vi "Entrain.vi"() -> ()   [LabVIEW 2012]
uses:
  <vilib>/Analysis/3filter.llb/Filter Passband Type.ctl
  Treatment.ctl
  Treatment type.ctl
  Data.ctl
  <vilib>/Platform/TimedLoop/XDataNode/timing_clust.ctl
  <vilib>/Platform/TimedLoop/XDataNode/nitl_modes.ctl
  <vilib>/Platform/TimedLoop/XDataNode/wakeup.ctl
  <vilib>/Platform/TimedLoop/XDataNode/XDataNode.xnode
  <vilib>/Platform/TimedLoop/XDataNode/XDNodeRunTimeDep.lvlib
  <vilib>/Analysis/NI_AALBase.lvlib
panel:
  out "R":dbl[](array[numeric])
  out "mean phase":dbl[](array[numeric])
  in  "reset phase":bool
  in  "enable":bool=TRUE caption="Enable motor"
  out "Cur freq":dbl caption="Stimulus frequency (Hz)"
  out "PSD":cluster{"f0":dbl, "df":dbl, "magnitude":dbl[]}[](graph)
  in  "Threshold":dbl=0.1
  out "Sweep":cluster{cluster{dbl, dbl}[]}[](graph)
  out "Raw data":waveform(dbl)[](graph)
  in  "Stop":bool
  in  "Go":bool
  in  "Treatment type":T1(tab)
  in  "Duration":dbl=inf min=0.0 step=1.0
  in  "Noise":dbl min=0.0 step=0.5
  in  "Frequency":dbl=1.0 min=0.0 step=0.05
  in  "Amplitude":dbl=30.0 min=0.0 step=1.0
  in  "Dur unit":enum16{"sec", "cycles"}(ring)
  in  "noise filter type":T2=enum."Bandpass"
  in  "Lo freq cutoff":dbl min=0.0 step=0.5
  in  "Hi freq cutoff":dbl min=0.0 step=0.5
  in  "End noise":dbl caption="End" min=0.0 step=0.5
  in  "End amplitude":dbl=30.0 caption="End" min=0.0 step=1.0
  in  "Start amp":dbl=30.0 caption="Start" min=0.0 step=1.0
  in  "Frequency":dbl=1.0 min=0.0 step=0.05
  in  "Start noise":dbl caption="Start" min=0.0 step=0.5
  in  "Lo freq cutoff 3":dbl caption="Lo freq cutoff" min=0.0 step=0.5
  in  "Hi freq cutoff 3":dbl caption="Hi freq cutoff" min=0.0 step=0.5
  in  "noise filter type 4":T2=enum."Bandpass" caption="Noise filter type"
  in  "Duration":dbl=inf min=0.0 step=1.0
  in  "Dur unit 4":enum16{"sec", "cycles"}(ring)
  in  "End freq":dbl=1.0 caption="End frequency" min=0.0 step=0.05
  in  "Duration":dbl=inf min=0.0 step=1.0
  in  "Noise":dbl min=0.0 step=0.5
  in  "Start freq":dbl=1.0 caption="Start frequency" min=0.0 step=0.05
  in  "Amp":dbl=30.0 caption="Amplitude" min=0.0 step=1.0
  in  "noise filter type 2":T2=enum."Bandpass" caption="Noise filter type"
  in  "Lo freq cutoff":dbl min=0.0 step=0.5
  in  "Hi freq cutoff":dbl min=0.0 step=0.5
  in  "Frequency 2":dbl=1.0 min=0.0 step=0.05
  in  "Amplitude 2":dbl=30.0 min=0.0 step=1.0
  in  "Duration":dbl=inf min=0.0 step=1.0
  in  "Frequency 1":dbl=1.0 min=0.0 step=0.05
  in  "Amplitude 1":dbl=30.0 min=0.0 step=1.0
  in  "Dur unit 2":enum16{"sec", "cycles"}(ring)
  out "Data file":path
  # "deg"
  # "Hz"
  # "deg"
  # "Hz"
  # "Hz"
  # "Noise is approximately\n4x lower than specified"
  # "Amplitude:"
  # "deg"
  # "Hz"
  # "deg"
  # "Hz"
  # "Hz"
  # "Send the position\nto zero"
  # "deg"
  # "Hz"
  # "Hz"
  # "deg"
  # "sec"
  # "deg"
  # "Hz"
  # "deg"
  # "Hz"
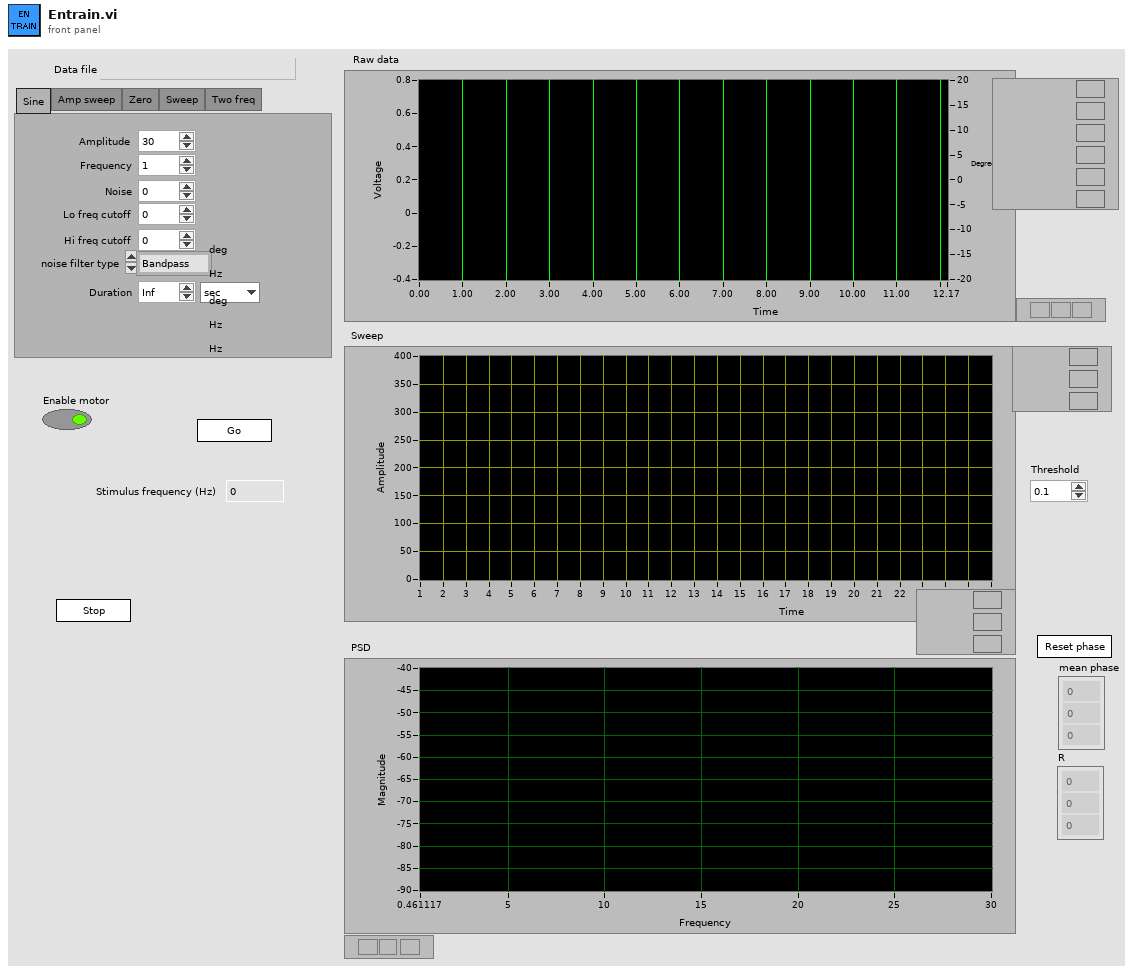
[diagram p1: front panel]
types:
  T1 = enum32{"Sine", "Amp sweep", "Zero", "Sweep", "Two freq"}
  T2 = typedef "NI_AALBase.lvlib/Filter Passband Type.ctl" = enum32{"Lowpass", "Highpass", "Bandpass", "Bandstop"}
  T3 = typedef "Treatment.ctl" = cluster{"sample":dbl, "startphase":dbl, "type":T4, "frequency":dbl, "amplitude":dbl, "noise":dbl, "duration":dbl, "kfreq":dbl, "noisehifreq":dbl, "frequency2":dbl, "amplitude2":dbl, "startphase2":dbl, "noise filter type":T2, "noiselofreq":dbl, "amp change":dbl, "noise change":dbl}
  T4 = typedef "Treatment type.ctl" = enum16{"Zero", "Sine", "Frequency sweep", "Two frequency"}
  T5 = typedef "Sampling info.ctl" = cluster{"Channels":T6[], "Sampling freq":i32, "Output freq":i32, "Update freq":i32, "Steps per rev":i32, "Counts per rev":i32, "Amplifier":string, "Motor driver":string, "Step bit":u8, "Max speed":dbl, "Max accel":dbl, "Pos gain":dbl, "Vel gain":dbl}
  T6 = typedef "Channel.ctl" = cluster{"Name":string, "Chan":tag, "Gain":u16, "Lo cutoff":dbl, "Hi cutoff":dbl, "Notch":bool}
  T7 = typedef "Data.ctl" = cluster{"Voltage data":dbl[][], "Encoder data":dbl[], "Motor output":dbl[], "Current treatment":T3, "Motor speed":dbl[], "Clipped motor":dbl[], "new treatment":bool}
  T8 = typedef "File refs.ctl" = cluster{"file":T9, "voltage data":i32, "motor data":i32, "command data":i32, "encoder data":i32}
  T9 = typedef "hid_t.ctl" = i32
  T10 = typedef "Run info.ctl" = cluster{"voltage task":refnum<k21>, "dummy output task":refnum<k21>, "digital output task":refnum<k21>, "encoder task":refnum<k21>, "n input samples":i32, "n output samples":i32, "max speed":dbl, "max accel":dbl, "last pos":dbl, "last vel":dbl, "pos gain":dbl, "vel gain":dbl, "input dt":dbl}
  T11 = typedef "XDNodeRunTimeDep.lvlib/timing_clust.ctl" = cluster{"Expected End [f-1]":u64, "Actual End [f-1]":u64, "Finished Late? [f-1]":bool, "Expected End [i-1]":u64, "Actual End [i-1]":u64, "Finished Late? [i-1]":bool, "Expected Start [i]":u64, "Actual Start [i]":u64, "Expected Start [f]":u64, "Actual Start [f]":u64, "Source Name":string, "Structure Name":string, "Period":i64, "Deadline":i64, "Offset":i64, "Start":i64, "Priority":i32, "Timeout":i32, "Mode":T12, "Wakeup Reason":T13, "Error":errorcluster, "Source Type":string, "Secondary Source Type":string, "Global End Time":u64, "Global Start Time":u64, "Frame Duration":u64, "Iteration Duration":u64, "Assigned CPU":i32, "I/O Scan Engine Mode":u32}
  T12 = typedef "XDNodeRunTimeDep.lvlib/nitl_modes.ctl" = enum32{"No Change", "Process missed periods, maintain original phase", "Discard missed periods, maintain original phase", "Process missed periods, ignore original phase", "Discard missed periods, ignore original phase"}
  T13 = typedef "XDNodeRunTimeDep.lvlib/wakeup.ctl" = enum32{"Normal", "Aborted", "Asynchronous wakeup", "Timing source error", "Timed loop error", "Timeout"}
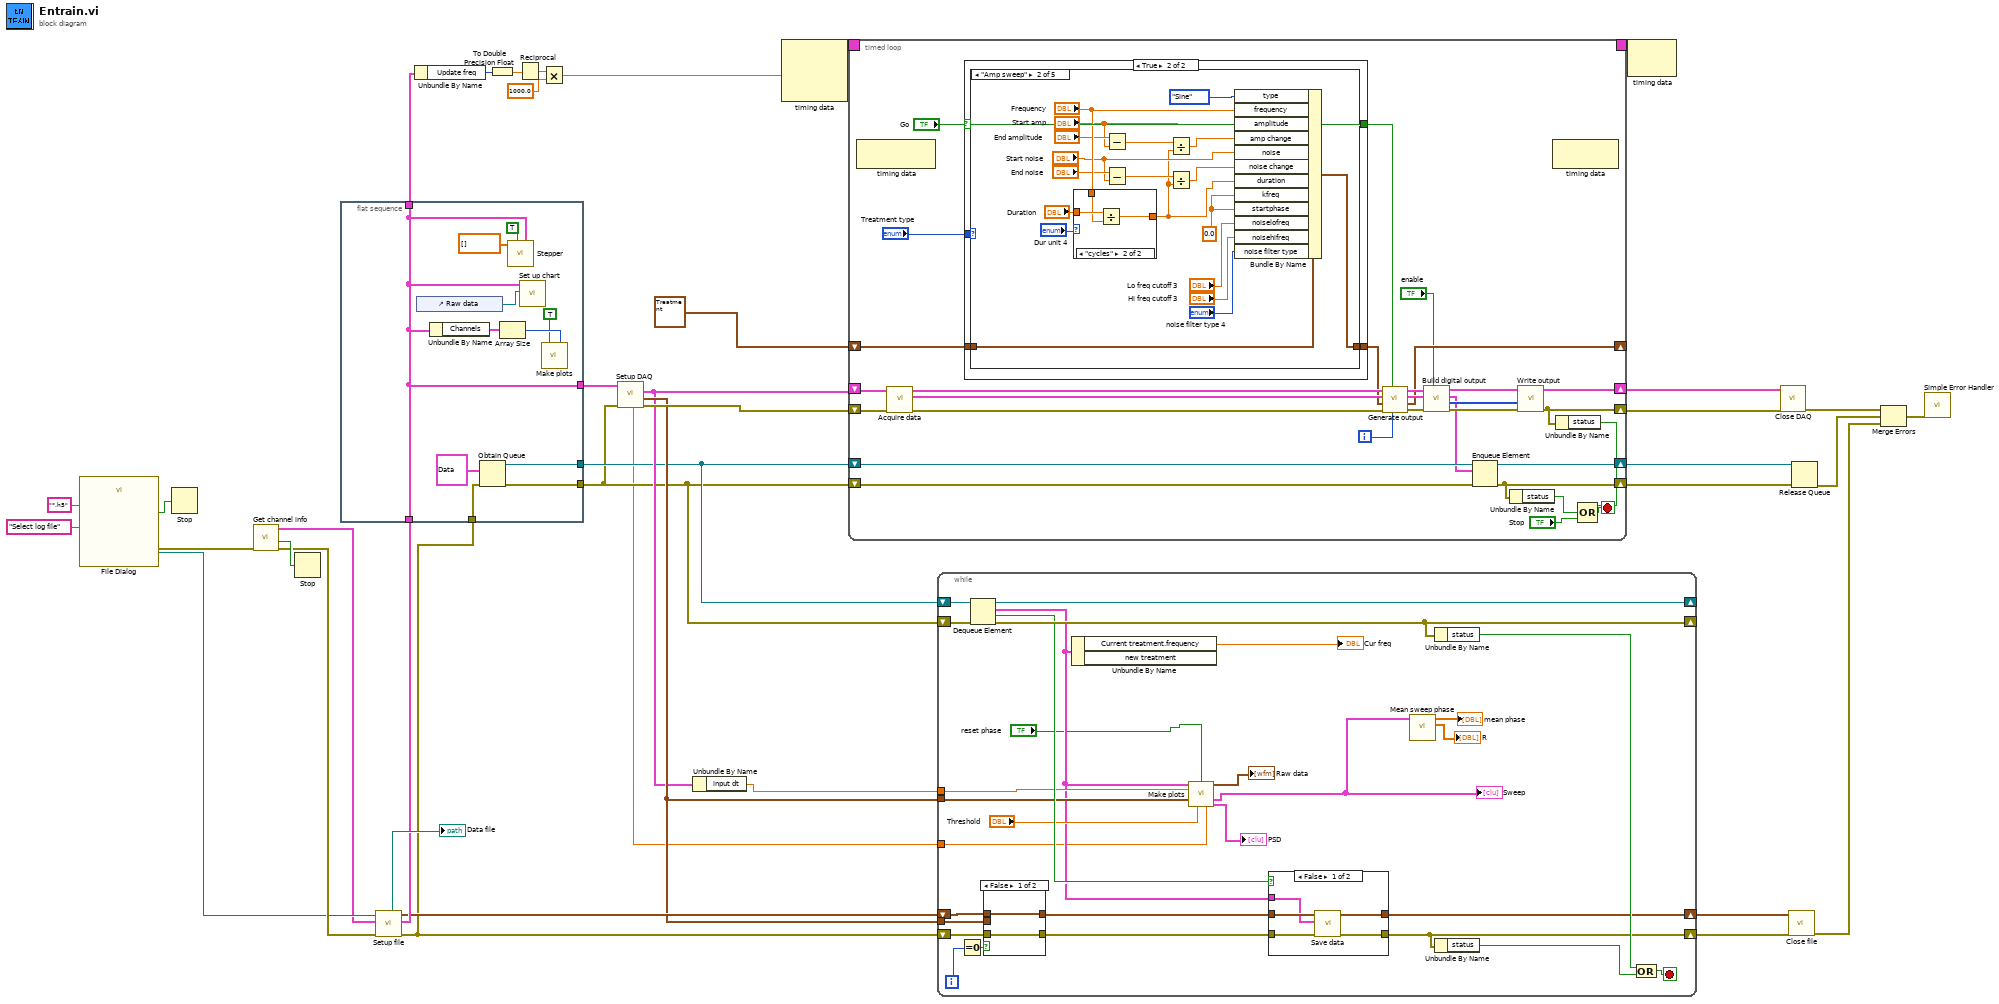
[diagram p0: block diagram]
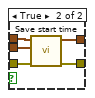
[diagram p2: hidden frame]
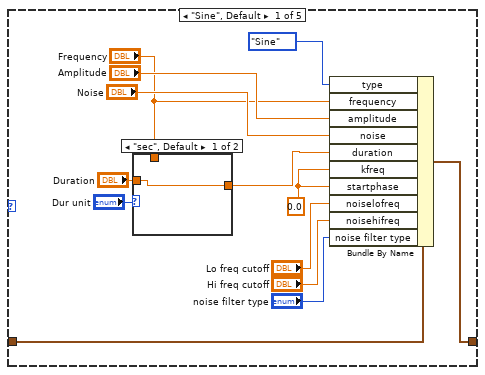
[diagram p5: hidden frame]
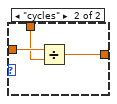
[diagram p6: hidden frame]
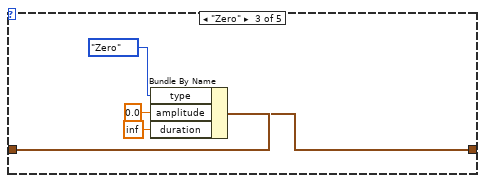
[diagram p8: hidden frame]
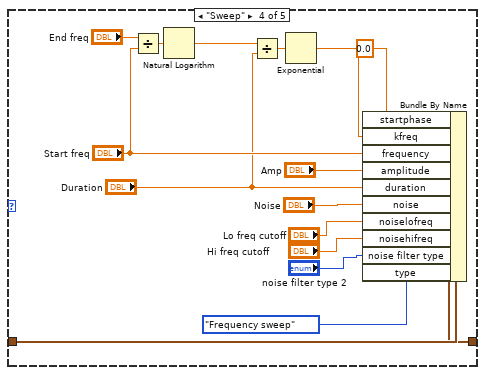
[diagram p9: hidden frame]
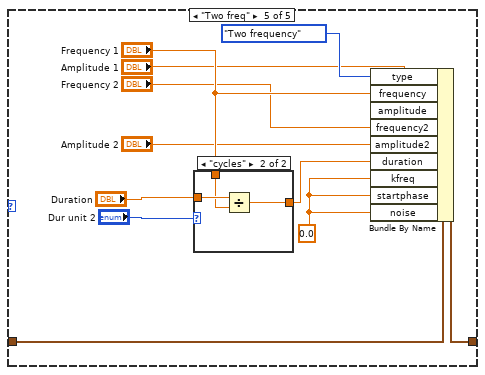
[diagram p10: hidden frame]
diagram:
  n1 = call "File Dialog"("prompt"="Select log file", "pattern (all files)"="*.h5") -> ("selected path"=w34:path, "cancelled"=w37:bool, "error out"=w33:errorcluster)  [unwired: 10 in, 1 out]
  n2 = Stop(stop? (T)=w37) -> ()
  n3 = call "Get channel info.vi"("error in"=w33) -> ("error out"=w35:errorcluster, "Cancelled"=w36:bool, "Sampling info"=w32:T5)  [unwired: 8 in]
  n4 = Stop(stop? (T)=w36) -> ()
  n5 = flat-sequence {
    tunnel: [w48] -> w3
    tunnel: w11 -> [w40]
    tunnel: [w42] -> w2
    tunnel: w9 -> [w41]
    tunnel: [w40] -> w7
    tunnel: [w40] -> w6
    frame #0 {
      n6 = control-ref of="Raw data"() -> (w46:refnum<vi>)
      n7 = Unbundle By Name(w40) -> ("Channels"=w45:T6[])
      n8 = Obtain Queue(element data type=T7 {"Voltage data"=[], "Encoder data"=[], "Motor output"=[], "Current treatment"={"sample"=0.0, "startphase"=0.0, "type"=enum."Zero", "frequency"=0.0, "amplitude"=0.0, "noise"=0.0, "duration"=0.0, "kfreq"=0.0, "noisehifreq"=0.0, "frequency2"=0.0, "amplitude2"=0.0, "startphase2"=0.0, "noise filter type"=enum."Lowpass", "noiselofreq"=0.0, "amp change"=0.0, "noise change"=0.0}, "Motor speed"=[], "Clipped motor"=[], "new treatment"=FALSE} ("Data"), error in (no error)=w41) -> (queue out=w48:refnum<queue>, error out=w42:errorcluster)  [unwired: 3 in, 1 out]
      n9 = Array Size(array=w45) -> (size(s)=w44:i32)
      n10 = call "Stepper.vi"("Sampling info"=w40, "initialize"=TRUE, "position"=dbl[] []) -> ()  [unwired: 7 in, 2 out]
      n11 = call "Set up chart.vi"("chart reference"=w46, "Sampling data"=w40) -> ()  [unwired: 10 in]
      n12 = call "Make plots.vi"("init"=TRUE, "nchan"=w44) -> ()  [unwired: 11 in, 3 out]
    }
  }
  n13 = call "Setup file.vi"("error in (no error)"=w35, "Sampling data"=w32, "selected path"=w34) -> ("error out"=w9:errorcluster, "Sampling data out"=w11:T5, "file refs"=w10:T8, "path out"=→"Data file":path)  [unwired: 5 in]
  n14 = Unbundle By Name(w7) -> ("Update freq"=w29:i32)
  n15 = To Double Precision Float(number=w29) -> (double precision float=w28:dbl)
  n16 = Reciprocal(x=w28) -> (1/x=w27:dbl)
  n17 = Multiply(x=w27, y=1000.0) -> (x*y=w14:dbl)
  n18 = call "Setup DAQ.vi"("error in (no error)"=w2, "Sampling info in"=w6) -> ("error out"=w13:errorcluster, "start time"=w8:timestamp, "Run info"=w4:T10, "output delay"=w1:dbl)  [unwired: 5 in, 1 out]
  n19 = Unbundle By Name(w4) -> ("input dt"=w12:dbl)
  n20 = node-c288(w14) -> (w31:T11)  [unwired: 2 in]
  n21 = timed-loop {
    timing: w31 -> [_]
    timing-out: [_] -> w30
    shift-right: [w58] -> _
    shift-left: T3 {"sample"=0.0, "startphase"=0.0, "type"=enum."Zero", "frequency"=0.0, "amplitude"=0.0, "noise"=0.0, "duration"=inf, "kfreq"=0.0, "noisehifreq"=20.0, "frequency2"=0.0, "amplitude2"=0.0, "startphase2"=0.0, "noise filter type"=enum."Lowpass", "noiselofreq"=0.0, "amp change"=0.0, "noise change"=0.0} ("Current treatment") -> [w54]
    shift-right: [w72] -> w17
    shift-left: w13 -> [w79]
    shift-right: [w71] -> w23
    shift-left: w2 -> [w74]
    shift-right: [w73] -> w16
    shift-left: w4 -> [w80]
    shift-right: [w66] -> w24
    shift-left: w3 -> [w75]
    i -> [w59]
    stop <- w68 stop-if-true
    n22 = node-c288() -> ()  [unwired: 1 in, 1 out]
    n23 = call "Acquire data.vi"("error in"=w79, "Run info"=w80) -> ("error out"=w76:errorcluster, "Data out"=w77:T7, "Run info out"=w78:T10)  [unwired: 7 in]
    n24 = case shown="True" "Go" {
      selector: "Go" -> [w81 w83]
      tunnel: "Treatment type" -> [_ w86]
      tunnel: w54 -> [w82 w85]
      tunnel: [w82 w84] -> w53
      tunnel: [w81 w83] -> w52
      frame False {
      }
      frame True {
        n25 = case shown="\"Amp sweep\"" w86 {
          tunnel: w85 -> [w93 w119 w128 w139 w154]
          tunnel: [w92 w118 w127 w138 w149] -> w84
          frame "Sine", Default {
            w90 = 0.0 ("kfreq")
            n26 = case shown="\"sec\", Default" "Dur unit" {
              tunnel: "Duration" -> [w100 w103]
              tunnel: "Frequency" -> [_ w102]
              tunnel: [w100 w101] -> w94
              frame "sec", Default {
              }
              frame "cycles" {
                n27 = Divide(x=w103, y=w102) -> (x/y=w101:dbl)
              }
            }
            n28 = Bundle By Name(cluster=w93, "type"=Treatment_type."Sine", "frequency"="Frequency", "amplitude"="Amplitude", "noise"="Noise", "duration"=w94, "kfreq"=w90, "startphase"=w90, "noiselofreq"="Lo freq cutoff", "noisehifreq"="Hi freq cutoff", "noise filter type"="noise filter type") -> (w92:T3)
          }
          frame "Amp sweep" {
            w116 = 0.0 ("kfreq")
            n29 = case shown="\"cycles\"" "Dur unit 4" {
              tunnel: "Duration" -> [w123 w126]
              tunnel: "Frequency" -> [_ w125]
              tunnel: [w123 w124] -> w105
              frame "sec", Default {
              }
              frame "cycles" {
                n30 = Divide(x=w126, y=w125) -> (x/y=w124:dbl)
              }
            }
            n31 = Subtract(x="End amplitude", y="Start amp") -> (x-y=w110:dbl)
            n32 = Subtract(x="End noise", y="Start noise") -> (x-y=w106:dbl)
            n33 = Divide(x=w110, y=w105) -> (x/y=w109:dbl)
            n34 = Divide(x=w106, y=w105) -> (x/y=w104:dbl)
            n35 = Bundle By Name(cluster=w119, "type"=Treatment_type."Sine", "frequency"="Frequency", "amplitude"="Start amp", "amp change"=w109, "noise"="Start noise", "noise change"=w104, "duration"=w105, "kfreq"=w116, "startphase"=w116, "noiselofreq"="Lo freq cutoff 3", "noisehifreq"="Hi freq cutoff 3", "noise filter type"="noise filter type 4") -> (w118:T3)
          }
          frame "Zero" {
            n36 = Bundle By Name(cluster=w128, "type"=Treatment_type."Zero", "amplitude"=0.0, "duration"=inf) -> (w127:T3)
          }
          frame "Sweep" {
            n37 = Divide(x="End freq", y="Start freq") -> (x/y=w147:dbl)
            n38 = Natural Logarithm(1:w147) -> (0:w146:dbl)
            n39 = Divide(x=w146, y="Duration") -> (x/y=w145:dbl)
            n40 = Exponential(1:w145) -> (0:w144:dbl)
            n41 = Bundle By Name(cluster=w139, "startphase"=0.0, "kfreq"=w144, "frequency"="Start freq", "amplitude"="Amp", "duration"="Duration", "noise"="Noise", "noiselofreq"="Lo freq cutoff", "noisehifreq"="Hi freq cutoff", "noise filter type"="noise filter type 2", "type"=Treatment_type."Frequency sweep") -> (w138:T3)
          }
          frame "Two freq" {
            w148 = 0.0 ("kfreq")
            n42 = case shown="\"cycles\"" "Dur unit 2" {
              tunnel: "Duration" -> [w159 w162]
              tunnel: "Frequency 1" -> [_ w161]
              tunnel: [w159 w160] -> w158
              frame "sec", Default {
              }
              frame "cycles" {
                n43 = Divide(x=w162, y=w161) -> (x/y=w160:dbl)
              }
            }
            n44 = Bundle By Name(cluster=w154, "type"=Treatment_type."Two frequency", "frequency"="Frequency 1", "amplitude"="Amplitude 1", "frequency2"="Frequency 2", "amplitude2"="Amplitude 2", "duration"=w158, "kfreq"=w148, "startphase"=w148, "noise"=w148) -> (w149:T3)
          }
        }
      }
    }
    n45 = call "Generate output.vi"("index"=w59, "new treatment"=w52, "error in"=w76, "Current treatment"=w53, "Data in"=w77, "Run info"=w78) -> ("error out"=w60:errorcluster, "Current treatment out"=w58:T3, "Data out"=w65:T7, "Run info out"=w63:T10)  [unwired: 2 in]
    n46 = call "Build digital output.vi"("enable"="enable", "error in"=w60, "Data in"=w65, "Run info"=w63) -> ("error out"=w61:errorcluster, "motor cmd"=w64:u32[], "Data out"=w57:T7, "Run info out"=w62:T10)  [unwired: 4 in]
    n47 = Enqueue Element(queue=w75, element=w57, error in (no error)=w74) -> (queue out=w66:refnum<queue>, error out=w71:errorcluster)  [unwired: 1 in, 1 out]
    n48 = Unbundle By Name(w71) -> ("status"=w69:bool)
    n49 = call "Write output.vi"("error in"=w61, "data"=w64, "Run info"=w62) -> ("error out"=w72:errorcluster, "Run info out"=w73:T10)  [unwired: 7 in]
    n50 = node-c288() -> ()  [unwired: 1 in, 1 out]
    n51 = Unbundle By Name(w72) -> ("status"=w70:bool)
    n52 = Compound Arithmetic op=OR(w70, w69, "Stop") -> (w68:bool)
  }
  n53 = while {
    shift-right: [w193] -> _
    shift-left: w2 -> [w187]
    shift-right: [w186] -> w22
    shift-left: w10 -> [w176]
    shift-right: [w185] -> w21
    shift-left: w9 -> [w174]
    shift-right: [w189] -> _
    shift-left: w3 -> [w188]
    tunnel: w8 -> [w183]
    tunnel: w12 -> [w181]
    tunnel: w8 -> [w179]
    tunnel: w1 -> [w169]
    i -> [w178]
    stop <- w192 stop-if-true
    n54 = Equal To 0?(x=w178) -> (x = 0?=w177:bool)
    n55 = Dequeue Element(queue=w188, error in (no error)=w187) -> (queue out=w189:refnum<queue>, element=w171:T7, timed out?=w184:bool, error out=w193:errorcluster)  [unwired: 1 in]
    n56 = case shown="False" w177 {
      tunnel: w179 -> [_ w200]
      tunnel: w176 -> [w195 w199]
      tunnel: [w195 w198] -> w175
      tunnel: w174 -> [w194 w197]
      tunnel: [w194 w196] -> w173
      frame False {
      }
      frame True {
        n57 = call "Save start time.vi"("error in (no error)"=w197, "Start time"=w200, "file refs"=w199) -> ("error out"=w196:errorcluster, "file refs out"=w198:T8)  [unwired: 7 in]
      }
    }
    n58 = Unbundle By Name(w171) -> ("Current treatment.frequency"=→"Cur freq":dbl)  [unwired: 1 out]
    n59 = call "Make plots.vi"("Data in"=w171, "reset phase"="reset phase", "dt"=w181, "start time"=w183, "threshold"="Threshold", "output delay"=w169) -> ("plot data"=→"Raw data":waveform(dbl)[], "Sweep data"=w168:cluster{cluster{dbl, dbl}[]}[], "PSD"=→"PSD":cluster{"f0":dbl, "df":dbl, "magnitude":dbl[]}[])  [unwired: 7 in]
    "Sweep" <- w168
    n60 = case shown="False" w184 {
      tunnel: w175 -> [w205 w207]
      tunnel: w173 -> [w204 w206]
      tunnel: w171 -> [w201 _]
      tunnel: [w203 w207] -> w186
      tunnel: [w202 w206] -> w185
      frame False {
        n61 = call "Save data.vi"("error in (no error)"=w204, "Data"=w201, "file refs"=w205) -> ("error out"=w202:errorcluster, "file refs out"=w203:T8)  [unwired: 7 in]
      }
      frame True {
      }
    }
    n62 = call "Mean sweep phase.vi"("Sweep data"=w168) -> ("R"=→"R":dbl[], "Mean phase"=→"mean phase":dbl[])  [unwired: 9 in]
    n63 = Unbundle By Name(w193) -> ("status"=w191:bool)
    n64 = Unbundle By Name(w185) -> ("status"=w190:bool)
    n65 = Compound Arithmetic op=OR(w191, w190) -> (w192:bool)
  }
  n66 = node-c288(w30) -> ()  [unwired: 1 out]
  n67 = call "Close DAQ.vi"("error in"=w17, "Run info"=w16) -> ("error out"=w15:errorcluster)  [unwired: 9 in]
  n68 = call "Close file.vi"("error in (no error)"=w21, "file refs"=w22) -> ("error out"=w19:errorcluster)  [unwired: 9 in]
  n69 = Release Queue(queue=w24, error in (no error)=w23) -> (error out=w20:errorcluster)  [unwired: 1 in, 2 out]
  n70 = Merge Errors(w15, w20, w19) -> (w18:errorcluster)
  n71 = call <vilib>:"Simple Error Handler.vi"("error in (no error)"=w18) -> ()  [unwired: 4 in, 5 out]
